vi "Questionable Temperature Event Enable.vi"(0 "VISA resource name":refnum<visa-resource-name>, 5 "Questionable Temperature Event Enable":T1, 11 "error in (no error)":errorcluster) -> (4 "VISA resource name out":refnum<visa-resource-name>, 15 "error out":errorcluster)   [LabVIEW 2018, in "XP Power PLS600.lvlib"]
doc: "Sets the value of the Questionable Temperatrure Enable register. This register is a mask for enabling specific bits from the Questionable Temperatrure Event register to set the questionable summary (QUES) bit of the Status Byte register. This bit (bit 3) is the logical OR of all the Questionable Event register bits that are enabled by the Questionable Status Enable registers.\n\nThe Questionable Temperature Event Enable consists of the following 2 bits:\n\nBit 0: Output Board Over-Temp\nBit 1: Primary Board Over-Temp"
uses:
  XP Power PLS600.lvlib
panel:
  # "Bit 0:  Output Board Over-Temp\nBit 1:  Primary Board Over-Temp"
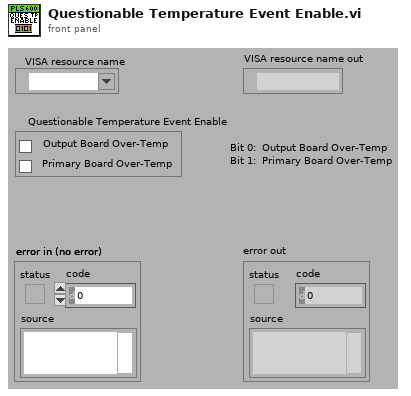
[diagram p1: front panel]
types:
  T1 = cluster{"Output Board Over-Temp":bool, "Primary Board Over-Temp":bool}
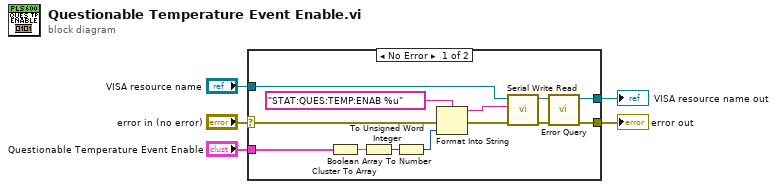
[diagram p0: block diagram]
diagram:
  n1 = case shown="No Error" "error in (no error)" {
    selector: "error in (no error)" -> [w18 w20]
    tunnel: "VISA resource name" -> [w11 w19]
    tunnel: [w6 w19] -> w5
    tunnel: [w7 w20] -> w4
    tunnel: "Questionable Temperature Event Enable" -> [w15 _]
    frame No Error {
      n2 = Cluster To Array(cluster=w15) -> (array=w16:bool[])
      n3 = Boolean Array To Number(Boolean array=w16) -> (number=w14:u32)
      n4 = To Unsigned Word Integer(number=w14) -> (unsigned 16bit integer=w13:u16)
      n5 = Format Into String(format string="STAT:QUES:TEMP:ENAB %u" ("Command to Send"), error in=w18, w13) -> (resulting string=w10:string, error out=w9:errorcluster)  [unwired: 1 in]
      n6 = call "Serial Write Read.vi"("error in (no error)"=w9, "Write Buffer"=w10, "VISA resource name"=w11) -> ("error out"=w8:errorcluster, "VISA resource name out"=w12:refnum<visa-resource-name>)  [unwired: 6 in, 1 out]
      n7 = call "Error Query.vi"("error in (no error)"=w8, "VISA resource name"=w12) -> ("error out"=w7:errorcluster, "VISA resource name out"=w6:refnum<visa-resource-name>)  [unwired: 6 in, 2 out]
    }
    frame Error {
    }
  }
  "error out" <- w4
  "VISA resource name out" <- w5
